vi "lights.vi"(8 "DO Channels":cluster{"DIO Pulse Pin":T1, "DIO Reset Pin":T1}={"DIO Pulse Pin"=enum."DIO 1", "DIO Reset Pin"=enum."DIO 1"}, 9 "PWM Channels":cluster{"Red":T2, "Green":T2, "Blue":T2}, 10 "AI Channels":cluster{"Audio Left":T3, "Audio Right":T3}={"Audio Left"=enum."AI 1", "Audio Right"=enum."AI 1"}) -> ()   [LabVIEW 2017]
uses:
  <vilib>/Rock Robotics/SystemInterfaces/AI/FPGA_AIChannel.ctl
  <vilib>/Rock Robotics/SystemInterfaces/DIO/FPGA_DIOPWMChannel.ctl
  <vilib>/Rock Robotics/SystemInterfaces/DIO/FPGA_DIOChannel.ctl
  modes.ctl
  State.ctl
  <vilib>/Rock Robotics/WPI/AnalogChannel/WPI_AnalogChannelDevRef.ctl
  <vilib>/Rock Robotics/WPI/PWM/WPI_PWMDeviceRef.ctl
  <vilib>/Rock Robotics/WPI/DigitalOutput/WPI_DigitalOutputDevRef.ctl
  <vilib>/addons/control/pid/pid.llb/PID EGU to Percentage (DBL).vi
  <vilib>/FRCT Team# 3937  Breakaway/Memory Library/memLib.lvlib
  <vilib>/addons/control/pid/NI_PID_pid.lvlib
panel:
  # "On Arduino Shield:\nAudio Left A0\nAudio Right A1\n\nStrob Pin D4\nReset Pin D5"
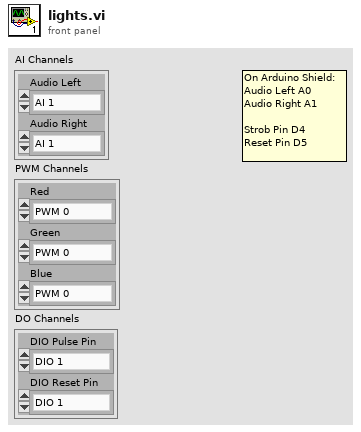
[diagram p1: front panel]
types:
  T1 = typedef "FPGA_DIOChannel.ctl" = enum8{"DIO 0", "DIO 1", "DIO 2", "DIO 3", "DIO 4", "DIO 5", "DIO 6", "DIO 7", "DIO 8", "DIO 9", "DIO MXP 0", "DIO MXP 1", "DIO MXP 2", "DIO MXP 3", "DIO MXP 4", "DIO MXP 5", "DIO MXP 6", "DIO MXP 7", "DIO MXP 8", "DIO MXP 9", "DIO MXP 10", "DIO MXP 11", "DIO MXP 12", "DIO MXP 13", "DIO MXP 14", "DIO MXP 15", "SPI Port CS1", "SPI Port CS2", "SPI Port CS3", "SPI Port MISO", "SPI Port MOSI", "Invalid"}
  T2 = typedef "FPGA_DIOPWMChannel.ctl" = enum8{"PWM 0", "PWM 1", "PWM 2", "PWM 3", "PWM 4", "PWM 5", "PWM 6", "PWM 7", "PWM 8", "PWM 9", "PWM MXP 0", "PWM MXP 1", "PWM MXP 2", "PWM MXP 3", "PWM MXP 4", "PWM MXP 5", "PWM MXP 6", "PWM MXP 7", "PWM MXP 8", "PWM MXP 9", "Invalid"}
  T3 = typedef "FPGA_AIChannel.ctl" = enum8{"AI 0", "AI 1", "AI 2", "AI 3", "AI MXP 0", "AI MXP 1", "AI MXP 2", "AI MXP 3", "Invalid"}
  T4 = typedef "State.ctl" = cluster{"Audio Left":T5, "Audio Right":T5, "Red":T6, "Green":T6, "Blue":T6, "Pulse Pin DevRef":T7, "Reset Pin DevRef":T7, "Audio Left Val":dbl, "Audio Right Val":dbl, "Red Val":dbl, "Green Val":dbl, "Blue Val":dbl}
  T5 = typedef "WPI_AnalogChannelDevRef.ctl" = cluster{"DevStatus":errorcluster, "Analog Channel":T3}
  T6 = typedef "WPI_PWMDeviceRef.ctl" = cluster{"DeviceStatus":errorcluster, "PWM Channel":T2}
  T7 = typedef "WPI_DigitalOutputDevRef.ctl" = cluster{"DIO Channel":T1, "DevStatus":errorcluster}
  T8 = typedef "modes.ctl" = enum16{"Init", "Setup", "Check Audio", "Set Lights"}
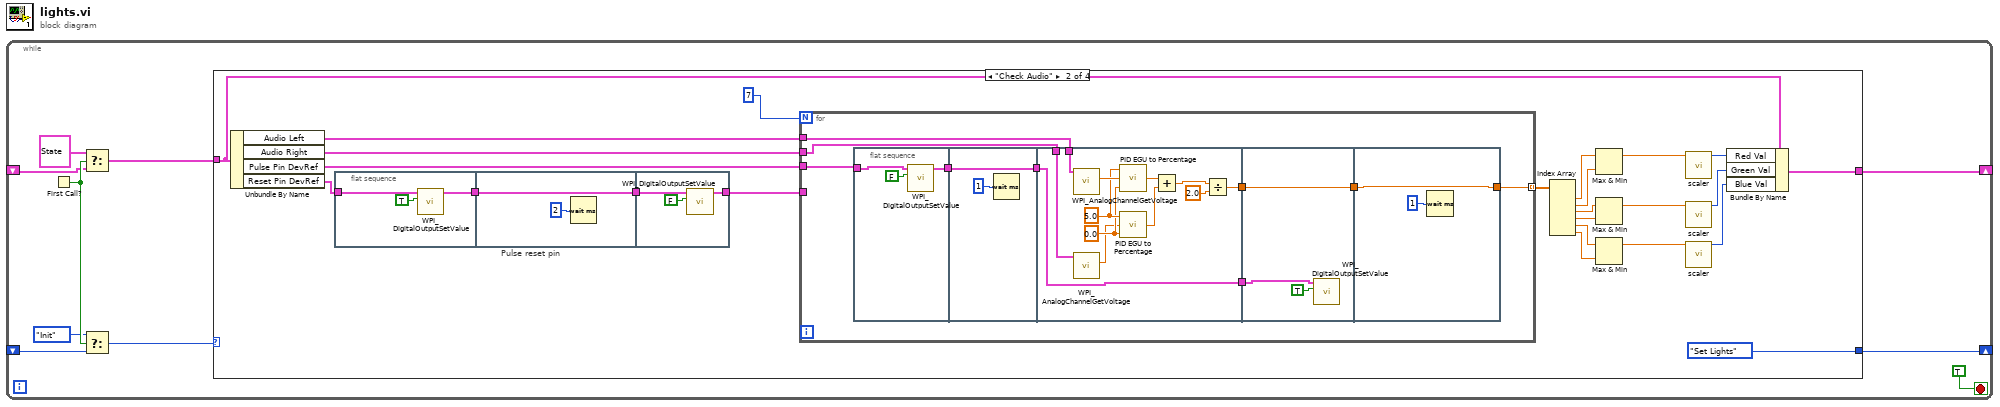
[diagram p0: block diagram]
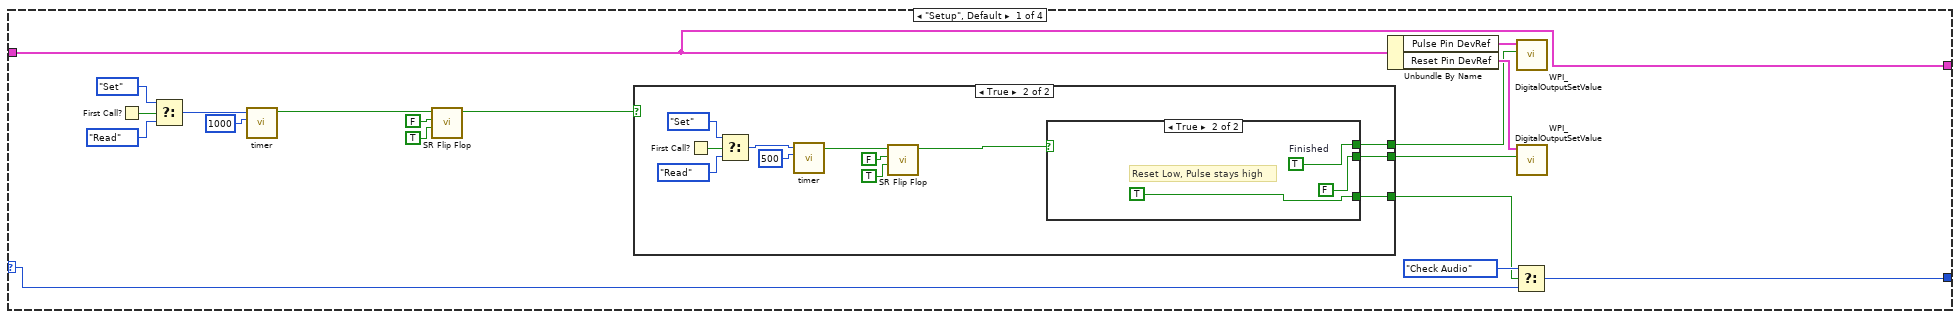
[diagram p2: hidden frame]
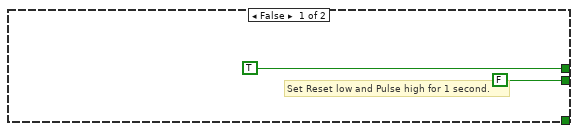
[diagram p3: hidden frame]
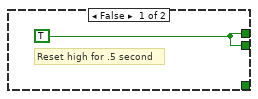
[diagram p4: hidden frame]
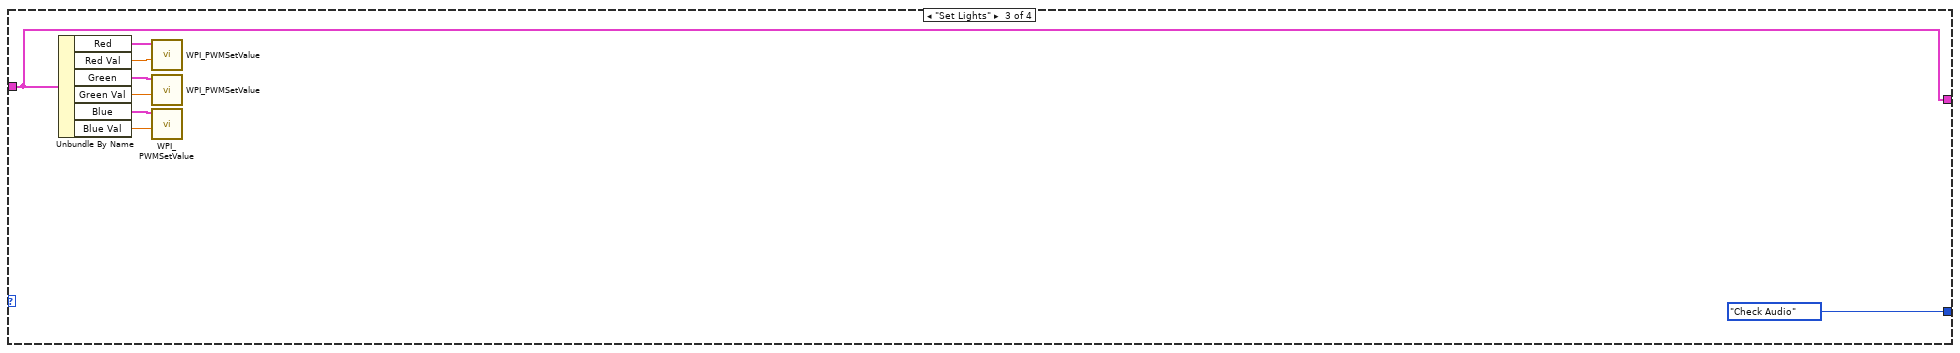
[diagram p5: hidden frame]
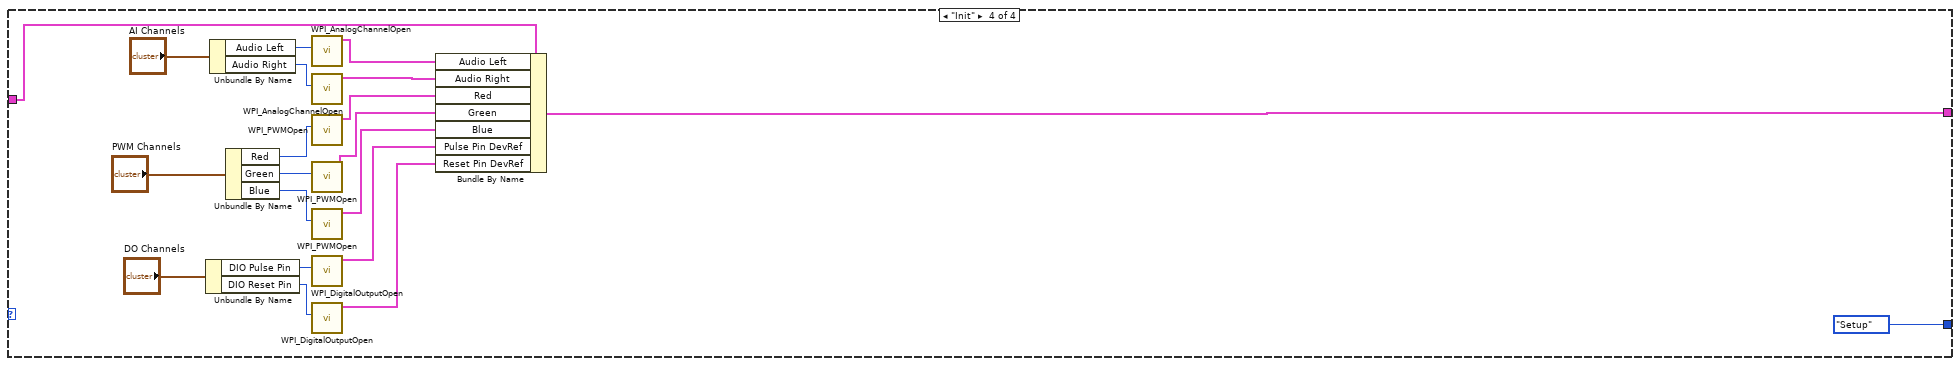
[diagram p6: hidden frame]
diagram:
  n1 = while {
    shift-right: [w6] -> _
    shift-left: _ -> [w5]
    shift-right: [w2] -> _
    shift-left: _ -> [w3]
    stop <- TRUE stop-if-true
    n2 = First Call?() -> (First Call?: T/F=w9:bool)
    n3 = Select(t=T4 {"Audio Left"={"DevStatus"={"status"=FALSE, "code"=0, "source"=""}, "Analog Channel"=enum."Invalid"}, "Audio Right"={"DevStatus"={"status"=FALSE, "code"=0, "source"=""}, "Analog Channel"=enum."Invalid"}, "Red"={"DeviceStatus"={"status"=FALSE, "code"=0, "source"=""}, "PWM Channel"=enum."PWM 0"}, "Green"={"DeviceStatus"={"status"=FALSE, "code"=0, "source"=""}, "PWM Channel"=enum."PWM 0"}, "Blue"={"DeviceStatus"={"status"=FALSE, "code"=0, "source"=""}, "PWM Channel"=enum."PWM 0"}, "Pulse Pin DevRef"={"DIO Channel"=enum."DIO 1", "DevStatus"={"status"=FALSE, "code"=0, "source"=""}}, "Reset Pin DevRef"={"DIO Channel"=enum."DIO 1", "DevStatus"={"status"=FALSE, "code"=0, "source"=""}}, "Audio Left Val"=0.0, "Audio Right Val"=0.0, "Red Val"=0.0, "Green Val"=0.0, "Blue Val"=0.0} ("Cluster"), s=w9, f=w5) -> (s? t:f=w7:T4)
    n4 = Select(t=modes."Init", s=w9, f=w3) -> (s? t:f=w10:T8)
    n5 = case shown="\"Check Audio\"" w10 {
      selector: w10 -> [w12 _ _ _]
      tunnel: w7 -> [w20 w70 w116 w137]
      tunnel: [w20 w53 w116 w136] -> w6
      tunnel: [w11 modes."Set Lights" modes."Check Audio" modes."Setup"] -> w2
      frame "Setup", Default {
        n6 = First Call?() -> (First Call?: T/F=w27:bool)
        n7 = Select(t=enum16{"Set", "Read"}."Set" ("Mode"), s=w27, f=enum16{"Set", "Read"}."Read") -> (s? t:f=w28:enum16{"Set", "Read"})
        n8 = call "timer.vi"("Target Time (ms)"=u32 1000, "Mode"=w28) -> ("Passed"=w23:bool)  [unwired: 9 in]
        n9 = call <vilib>:"SR Flip Flop.vi"("Enable"=TRUE, "Reset"=FALSE, "Set"=w23) -> ("Output"=w17:bool)  [unwired: 8 in]
        n10 = case shown="True" w17 {
          tunnel: [TRUE w32] -> w15
          tunnel: [FALSE w37] -> w16
          tunnel: [_ w31] -> w13
          frame False {
            # "Set Reset low and Pulse high for 1 second."
          }
          frame True {
            n11 = First Call?() -> (First Call?: T/F=w38:bool)
            n12 = Select(t=enum16{"Set", "Read"}."Set" ("Mode"), s=w38, f=enum16{"Set", "Read"}."Read") -> (s? t:f=w42:enum16{"Set", "Read"})
            n13 = call "timer.vi"("Target Time (ms)"=u32 500, "Mode"=w42) -> ("Passed"=w34:bool)  [unwired: 9 in]
            n14 = call <vilib>:"SR Flip Flop.vi"("Enable"=TRUE, "Reset"=FALSE, "Set"=w34) -> ("Output"=w33:bool)  [unwired: 8 in]
            n15 = case shown="True" w33 {
              tunnel: [w43 FALSE] -> w37
              tunnel: [w43 w45] -> w32
              tunnel: [_ TRUE] -> w31
              frame False {
                w43 = TRUE
                # "Reset high for .5 second"
              }
              frame True {
                w45 = TRUE  # Finished
                # "Reset Low, Pulse stays high"
              }
            }
          }
        }
        n16 = Unbundle By Name(w20) -> ("Pulse Pin DevRef"=w19:T7, "Reset Pin DevRef"=w18:T7)
        n17 = Select(t=modes."Check Audio", s=w13, f=w12) -> (s? t:f=w11:T8)
        n18 = call <vilib>:"WPI_DigitalOutputSetValue.vi"("Value"=w15, "DigitalOutputDevRef"=w19) -> ()  [unwired: 8 in, 2 out]
        n19 = call <vilib>:"WPI_DigitalOutputSetValue.vi"("Value"=w16, "DigitalOutputDevRef"=w18) -> ()  [unwired: 8 in, 2 out]
      }
      frame "Check Audio" {
        n20 = Unbundle By Name(w70) -> ("Audio Left"=w63:T5, "Audio Right"=w62:T5, "Pulse Pin DevRef"=w65:T7, "Reset Pin DevRef"=w68:T7)
        n21 = flat-sequence "Pulse reset pin" {
          tunnel: w68 -> [w73]
          tunnel: [w71] -> w66
          tunnel: [w74] -> w67
          tunnel: w66 -> [w74]
          tunnel: w67 -> [w77]
          tunnel: [w76] -> w64
          frame #0 {
            n22 = call <vilib>:"WPI_DigitalOutputSetValue.vi"("Value"=TRUE, "DigitalOutputDevRef"=w73) -> ("DigitalOutputDevRef"=w71:T7)  [unwired: 8 in, 1 out]
          }
          frame #1 {
            n23 = Wait (ms)(milliseconds to wait=u32 2) -> ()  [unwired: 1 out]
          }
          frame #2 {
            n24 = call <vilib>:"WPI_DigitalOutputSetValue.vi"("Value"=FALSE, "DigitalOutputDevRef"=w77) -> ("DigitalOutputDevRef"=w76:T7)  [unwired: 8 in, 1 out]
          }
        }
        n25 = for {
          N: 7 -> [_]
          tunnel: w65 -> [w87]
          tunnel: w64 -> [_]
          tunnel: w63 -> [w86]
          tunnel: w62 -> [w85]
          tunnel: [w79] -> w61 mode=indexing
          n26 = flat-sequence {
            tunnel: w87 -> [w90]
            tunnel: [w88] -> w81
            tunnel: [w91] -> w82
            tunnel: w81 -> [w91]
            tunnel: w86 -> [w104]
            tunnel: w85 -> [w103]
            tunnel: [w94] -> w84
            tunnel: [w93] -> w83
            tunnel: w82 -> [w93]
            tunnel: w84 -> [w107]
            tunnel: w83 -> [w105]
            tunnel: [w107] -> w80
            tunnel: [w109] -> w79
            tunnel: w80 -> [w109]
            frame #0 {
              n27 = call <vilib>:"WPI_DigitalOutputSetValue.vi"("Value"=FALSE, "DigitalOutputDevRef"=w90) -> ("DigitalOutputDevRef"=w88:T7)  [unwired: 8 in, 1 out]
            }
            frame #1 {
              n28 = Wait (ms)(milliseconds to wait=u32 1) -> ()  [unwired: 1 out]
            }
            frame #2 {
              w100 = 0.0 ("minimum (EGU)")
              w101 = 5.0 ("maximum (EGU)")
              n29 = call <vilib>:"WPI_AnalogChannelGetVoltage.vi"("AIDeviceRef"=w104) -> ("Voltage"=w102:dbl)  [unwired: 8 in, 2 out]
              n30 = call <vilib>:"WPI_AnalogChannelGetVoltage.vi"("AIDeviceRef"=w103) -> ("Voltage"=w99:dbl)  [unwired: 8 in, 2 out]
              n31 = call-poly <vilib>:"PID EGU to Percentage.vi"("minimum (EGU)"=w100, "input (EGU)"=w102, "maximum (EGU)"=w101) -> ("% span"=w98:dbl)
              n32 = call-poly <vilib>:"PID EGU to Percentage.vi"("minimum (EGU)"=w100, "input (EGU)"=w99, "maximum (EGU)"=w101) -> ("% span"=w97:dbl)
              n33 = Add(x=w98, y=w97) -> (x+y=w96:dbl)
              n34 = Divide(x=w96, y=2.0) -> (x/y=w94:dbl)
            }
            frame #3 {
              n35 = call <vilib>:"WPI_DigitalOutputSetValue.vi"("Value"=TRUE, "DigitalOutputDevRef"=w105) -> ()  [unwired: 8 in, 2 out]
            }
            frame #4 {
              n36 = Wait (ms)(milliseconds to wait=u32 1) -> ()  [unwired: 1 out]
            }
          }
        }
        n37 = Index Array(array=w61) -> (element #1=w60:dbl, element #2=w59:dbl, element #3=w48:dbl, element #4=w47:dbl, element #5=w51:dbl, element #6=w50:dbl)  [unwired: 6 in]
        n38 = Max & Min(x=w60, y=w59) -> (max(x,y)=w58:dbl)  [unwired: 1 out]
        n39 = Max & Min(x=w48, y=w47) -> (max(x,y)=w49:dbl)  [unwired: 1 out]
        n40 = Max & Min(x=w51, y=w50) -> (max(x,y)=w55:dbl)  [unwired: 1 out]
        n41 = call "scaler.vi"("Input"=w58) -> ("Output"=w57:u8)  [unwired: 10 in]
        n42 = call "scaler.vi"("Input"=w49) -> ("Output"=w56:u8)  [unwired: 10 in]
        n43 = call "scaler.vi"("Input"=w55) -> ("Output"=w54:u8)  [unwired: 10 in]
        n44 = Bundle By Name(cluster=w70, "Red Val"=w57, "Green Val"=w56, "Blue Val"=w54) -> (w53:T4)
      }
      frame "Set Lights" {
        n45 = Unbundle By Name(w116) -> ("Red"=w115:T6, "Red Val"=w114:dbl, "Green"=w113:T6, "Green Val"=w112:dbl, "Blue"=w111:T6, "Blue Val"=w110:dbl)
        n46 = call <vilib>:"WPI_PWMSetValue.vi"("Value"=w114, "PWMDeviceRef"=w115) -> ()  [unwired: 8 in, 2 out]
        n47 = call <vilib>:"WPI_PWMSetValue.vi"("Value"=w112, "PWMDeviceRef"=w113) -> ()  [unwired: 8 in, 2 out]
        n48 = call <vilib>:"WPI_PWMSetValue.vi"("Value"=w110, "PWMDeviceRef"=w111) -> ()  [unwired: 8 in, 2 out]
      }
      frame "Init" {
        n49 = Unbundle By Name("DO Channels") -> ("DIO Pulse Pin"=w119:T1, "DIO Reset Pin"=w118:T1)
        n50 = Unbundle By Name("AI Channels") -> ("Audio Left"=w126:T3, "Audio Right"=w125:T3)
        n51 = Unbundle By Name("PWM Channels") -> ("Red"=w123:T2, "Green"=w122:T2, "Blue"=w121:T2)
        n52 = call <vilib>:"WPI_AnalogChannelOpen.vi"("Analog Channel"=w126) -> ("AIDeviceRef"=w135:T5)  [unwired: 9 in, 1 out]
        n53 = call <vilib>:"WPI_AnalogChannelOpen.vi"("Analog Channel"=w125) -> ("AIDeviceRef"=w134:T5)  [unwired: 9 in, 1 out]
        n54 = call <vilib>:"WPI_PWMOpen.vi"("PWM Channel"=w123) -> ("PWMDeviceRef"=w133:T6)  [unwired: 9 in, 1 out]
        n55 = call <vilib>:"WPI_PWMOpen.vi"("PWM Channel"=w122) -> ("PWMDeviceRef"=w132:T6)  [unwired: 9 in, 1 out]
        n56 = call <vilib>:"WPI_PWMOpen.vi"("PWM Channel"=w121) -> ("PWMDeviceRef"=w131:T6)  [unwired: 9 in, 1 out]
        n57 = call <vilib>:"WPI_DigitalOutputOpen.vi"("DIO Channel"=w119) -> ("DigitalOutputDevRef"=w130:T7)  [unwired: 9 in, 1 out]
        n58 = call <vilib>:"WPI_DigitalOutputOpen.vi"("DIO Channel"=w118) -> ("DigitalOutputDevRef"=w129:T7)  [unwired: 9 in, 1 out]
        n59 = Bundle By Name(cluster=w137, "Audio Left"=w135, "Audio Right"=w134, "Red"=w133, "Green"=w132, "Blue"=w131, "Pulse Pin DevRef"=w130, "Reset Pin DevRef"=w129) -> (w136:T4)
      }
    }
  }
